vi "Error Reported.vi"(8 "error in (no error)":errorcluster, 9 "Additional Information":string, 10 "Error":errorcluster) -> (0 "error out":errorcluster)   [LabVIEW 2020, in "Launcher.lvlib"]
doc: "Send the Error Reported event to any VI registered to listen to events from the owning module.\n_____\nBased on Delacor QMH Project Template 5.0.0.82."
uses:
  Launcher.lvlib
  Error Reported Argument--cluster.ctl
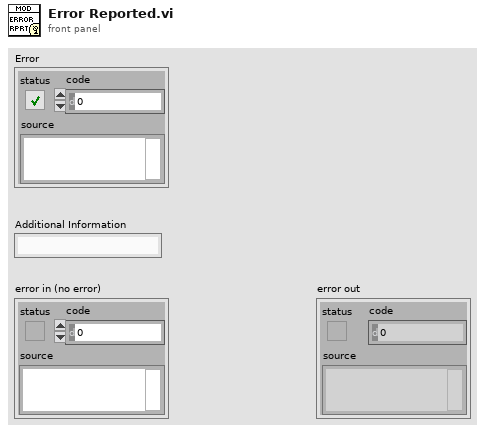
[diagram p1: front panel]
types:
  T1 = typedef "Launcher.lvlib/Error Reported Argument--cluster.ctl" = cluster{"Error":errorcluster, "Additional Information":string, "Module Name":string}
  T2 = typedef "Launcher.lvlib/Broadcast Events--cluster.ctl" = cluster{"Module Did Init":refnum<user-event>, "Status Updated":refnum<user-event>, "Error Reported":refnum<user-event>, "Module Did Stop":refnum<user-event>, "Update Module Execution Status":refnum<user-event>}
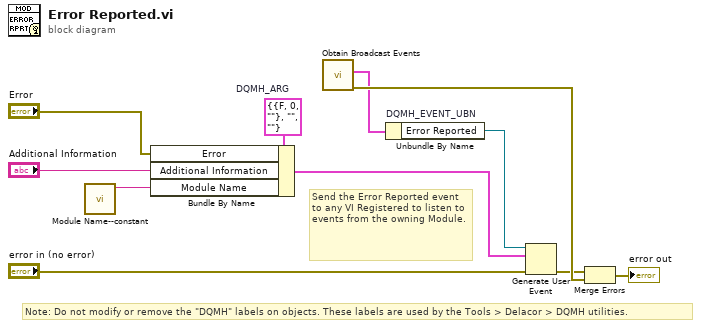
[diagram p0: block diagram]
diagram:
  w4 = T1 {"Error"={"status"=FALSE, "code"=0, "source"=""}, "Additional Information"="", "Module Name"=""}  # DQMH_ARG
  # "Note: Do not modify or remove the \"DQMH\" labels on objects. These labels are used by the Tools > Delacor > DQMH utilities."
  # "Send the Error Reported event to any VI Registered to listen to events from the owning Module."
  n1 = call "Module Name--constant.vi"() -> ("Module Name"=w1:string)  [unwired: 11 in]
  n2 = Bundle By Name(cluster=w4, "Error"="Error", "Additional Information"="Additional Information", "Module Name"=w1) -> (w3:T1)
  n3 = call "Obtain Broadcast Events.vi"() -> ("error out"=w8:errorcluster, "Launcher Broadcast Events"=w6:T2)  [unwired: 10 in]
  n4 = Unbundle By Name "DQMH_EVENT_UBN"(w6) -> ("Error Reported"=w5:refnum<user-event>)
  n5 = Generate User Event(user event=w5, event data cluster=w3, error in="error in (no error)") -> (error out=w7:errorcluster)  [unwired: 1 in, 1 out]
  n6 = Merge Errors(w7, w8) -> (→"error out":errorcluster)
